vi "Initialize Settings 1.0.vi"(8 "error in (no error)":errorcluster, 11 "settings 1.0":cluster{"key":string, "value":string}[](array[cluster])) -> (0 "error out":errorcluster, 3 "configuration 1.0":T1)   [LabVIEW 2017, in "DSF Core.lvlib" / "Group Configuration.lvclass"]
uses:
  Group Configuration.lvclass
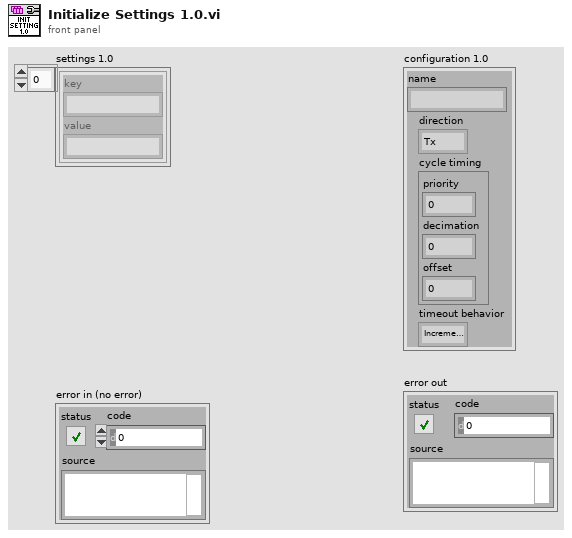
[diagram p1: front panel]
types:
  T1 = cluster{"name":string, "direction":enum8{"Tx", "Rx"}, "cycle timing":cluster{"priority":u64, "decimation":u64, "offset":u64}, "timeout behavior":enum8{"Increment Late Count", "Throw Error"}}
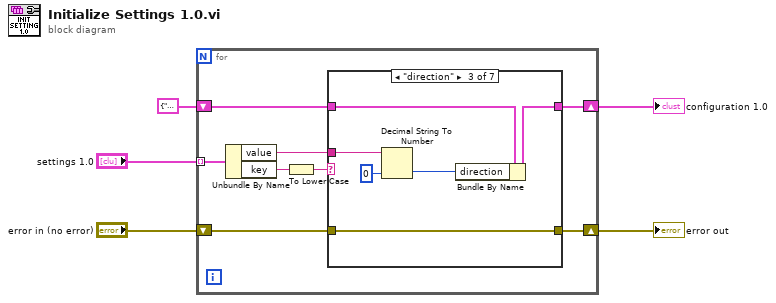
[diagram p0: block diagram]
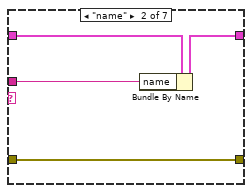
[diagram p3: hidden frame]
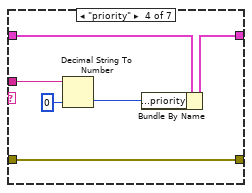
[diagram p4: hidden frame]
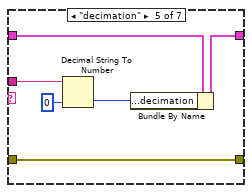
[diagram p5: hidden frame]
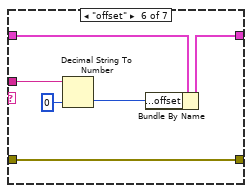
[diagram p6: hidden frame]
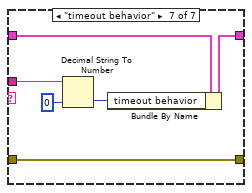
[diagram p7: hidden frame]
diagram:
  n1 = for {
    shift-right: [w8] -> w2
    shift-left: T1 {"name"="Group", "direction"=enum."Tx", "cycle timing"={"priority"=100, "decimation"=1, "offset"=0}, "timeout behavior"=enum."Increment Late Count"} ("configuration") -> [w9]
    tunnel: "settings 1.0" -> [w13] mode=indexing
    shift-right: [w6] -> w5
    shift-left: "error in (no error)" -> [w7]
    n2 = Unbundle By Name(w13) -> ("value"=w10:string, "key"=w12:string)
    n3 = To Lower Case(string=w12) -> (all lower case string=w11:string)
    n4 = case shown="\"direction\"" w11 {
      tunnel: w10 -> [_ w17 w21 w27 w33 w39 w45]
      tunnel: w9 -> [w15 w19 w25 w31 w37 w43 w49]
      tunnel: [w15 w18 w24 w30 w36 w42 w48] -> w8
      tunnel: w7 -> [w14 w16 w23 w29 w35 w41 w47]
      tunnel: [w14 w16 w23 w29 w35 w41 w47] -> w6
      frame Default {
        # "Unknown setting."
      }
      frame "name" {
        n5 = Bundle By Name(cluster=w19, "name"=w17) -> (w18:T1)
      }
      frame "direction" {
        n6 = Decimal String To Number(string=w21, default (0L)=u8 0 ("default (0 I32)")) -> (number=w22:u8)  [unwired: 1 in, 1 out]
        n7 = Bundle By Name(cluster=w25, "direction"=w22) -> (w24:T1)
      }
      frame "priority" {
        n8 = Decimal String To Number(string=w27, default (0L)=u64 0 ("default (0 I32)")) -> (number=w28:u64)  [unwired: 1 in, 1 out]
        n9 = Bundle By Name(cluster=w31, "cycle timing.priority"=w28) -> (w30:T1)
      }
      frame "decimation" {
        n10 = Decimal String To Number(string=w33, default (0L)=u64 0 ("default (0 I32)")) -> (number=w34:u64)  [unwired: 1 in, 1 out]
        n11 = Bundle By Name(cluster=w37, "cycle timing.decimation"=w34) -> (w36:T1)
      }
      frame "offset" {
        n12 = Decimal String To Number(string=w39, default (0L)=u64 0 ("default (0 I32)")) -> (number=w40:u64)  [unwired: 1 in, 1 out]
        n13 = Bundle By Name(cluster=w43, "cycle timing.offset"=w40) -> (w42:T1)
      }
      frame "timeout behavior" {
        n14 = Decimal String To Number(string=w45, default (0L)=u8 0 ("default (0 I32)")) -> (number=w46:u8)  [unwired: 1 in, 1 out]
        n15 = Bundle By Name(cluster=w49, "timeout behavior"=w46) -> (w48:T1)
      }
    }
  }
  "error out" <- w5
  "configuration 1.0" <- w2
